vi "Switch Flatten Test Parameters.vi"(7 "Test Configuration (\"\")":string, 9 "error in (no error)":errorcluster, 10 "Parameter Variant":variant) -> (1 "error out":errorcluster, 2 "Parameter String":string)   [LabVIEW 2011]
uses:
  TypeDefs/Switch Test Parameters.ctl
  TypeDefs/Switch Stimulus Parameters.ctl
  TypeDefs/Switch Type.ctl
  TypeDefs/Switch Instrument Info.ctl
  Switch Version.vi
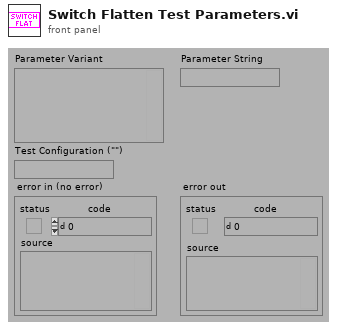
[diagram p1: front panel]
types:
  T1 = typedef "Switch Test Parameters.ctl" = cluster{"Stimulus":T2, "Switch Info":T4}
  T2 = typedef "Switch Stimulus Parameters.ctl" = cluster{"Blank Screen":bool, "SWI Position":variant, "Switch Type":T3}
  T3 = typedef "Switch Type.ctl" = enum16{"Sea-Level", "Simulator", "SI-0206-SW", "SI-0309-SW", "SI-0310-SW", "Front End"}
  T4 = typedef "Switch Instrument Info.ctl" = cluster{"sDriverId":string, "sDriverType":string, "Model":string, "Serial":string, "USB Serial":string}
  T5 = typedef "OGAB Version.ctl" = cluster{"Version":string, "Build Number":u32, "Build Date/Time":dbl}
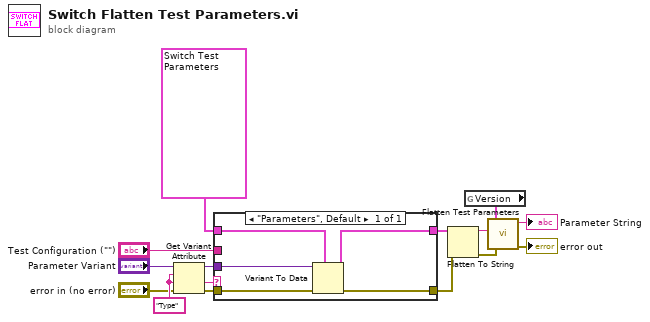
[diagram p0: block diagram]
diagram:
  w14 = "Type" ("name")
  n1 = Get Variant Attribute(Variant="Parameter Variant", name=w14, default value (empty Variant)=w14, error in="error in (no error)") -> (duplicate Variant=w3:variant, value=w2:string, error out=w7:errorcluster)  [unwired: 1 out]
  n2 = case shown="\"Parameters\", Default" w2 {
    tunnel: w3 -> [w20]
    tunnel: T1 {"Stimulus"={"Blank Screen"=FALSE, "SWI Position"=variant, "Switch Type"=enum."Sea-Level"}, "Switch Info"={"sDriverId"="", "sDriverType"="", "Model"="", "Serial"="", "USB Serial"=""}} ("DCA Test Parameters") -> [w16]
    tunnel: [w17] -> w1
    tunnel: [w19] -> w4
    tunnel: w7 -> [w18]
    tunnel: "Test Configuration (\"\")" -> [_]
    frame "Parameters", Default {
      n3 = Variant To Data(error in=w18, type=w16, Variant=w20) -> (data=w17:T1, error out=w19:errorcluster)
    }
  }
  n4 = Flatten To String(anything=w1, error in (no error)=w4) -> (data string=w13:string, error out=w11:errorcluster)  [unwired: 3 out]
  n5 = global read "Switch Version.vi" "Version"() -> (w12:T5)
  n6 = call "Flatten Test Parameters.vi"("error in (no error)"=w11, "Flattened Test Parameters (\"\")"=w13, "Test Version"=w12) -> ("error out"=→"error out":errorcluster, "Flattened Test Parameters with Version"=→"Parameter String":string)  [unwired: 3 out]
